vi "Configure Services.vi"(8 "error in":errorcluster, 10 "Entity Manager":refnum<class "Entity Manager.lvclass">, 11 "HTTP Server In":refnum<class "Server.lvclass">) -> (0 "error out":errorcluster, 3 "HTTP Server":refnum<class "Server.lvclass">)   [LabVIEW 2022 SP3, in "HTTP-Conditum.lvlib"]
doc: "<b>Configure Services.vi</b> is used insetad of <b>Configure Auth.vi</b> when a user entity is not used for authentication mechanisms. This VI wraps the specified entity manager instance in a HTTP service to be accessible within http requests.\n\nBefore calling this VI, all used entities should be registered with the entity manager instance for best performance."
uses:
  HTTP-Conditum.lvlib
  <vilib>/IlluminatedG/IG HTTP Server/HTTP Server/Server/Server.lvclass
  <vilib>/IlluminatedG/IG Conditum/Conditum/Entity Manager/Entity Manager.lvclass
  Entity Manager Service/Entity Manager Service.lvclass
  C:/Program Files (x86)/National Instruments/LabVIEW 2022/vi.lib/IlluminatedG/IG HTTP Server/HTTP Server/Service/Service.lvclass
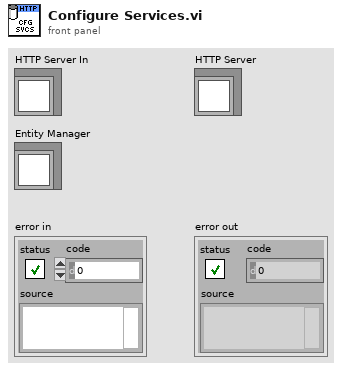
[diagram p1: front panel]
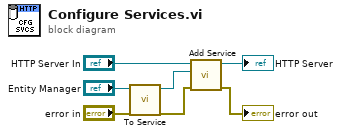
[diagram p0: block diagram]
diagram:
  n1 = call "To Service.vi"("Entity Manager"="Entity Manager") -> ("Entity Manager Service"=w4:refnum<class "Entity Manager Service.lvclass">)  [unwired: 10 in]
  n2 = call <vilib>:"Add Service.vi"("error in (no error)"="error in", "Service"=w4, "Server in"="HTTP Server In") -> ("error out"=→"error out":errorcluster, "Server out"=→"HTTP Server":refnum<class "Server.lvclass">)  [unwired: 7 in]
